vi "Ysingle.vi"(8 "error in (no error)":errorcluster, 11 "MagSpecCamera in":refnum<class "MagSpecCamera.lvclass">) -> (0 "error out":errorcluster, 3 "MagSpecCamera in":refnum<class "MagSpecCamera.lvclass">)   [LabVIEW 2020, in "MagSpecCamera.lvclass"]
uses:
  MagSpecCamera.lvclass
  finalCalib--Cluster.ctl
  MagSpecCamera.lvclass/MagSpecCamera.ctl
  NI_AALBase.lvlib
panel:
  out "Working":i32[](array[numeric])
  out "GOOD - not working":i32[](array[numeric])
  out "pixel angle (y)(pixel)":dbl[][](graph)
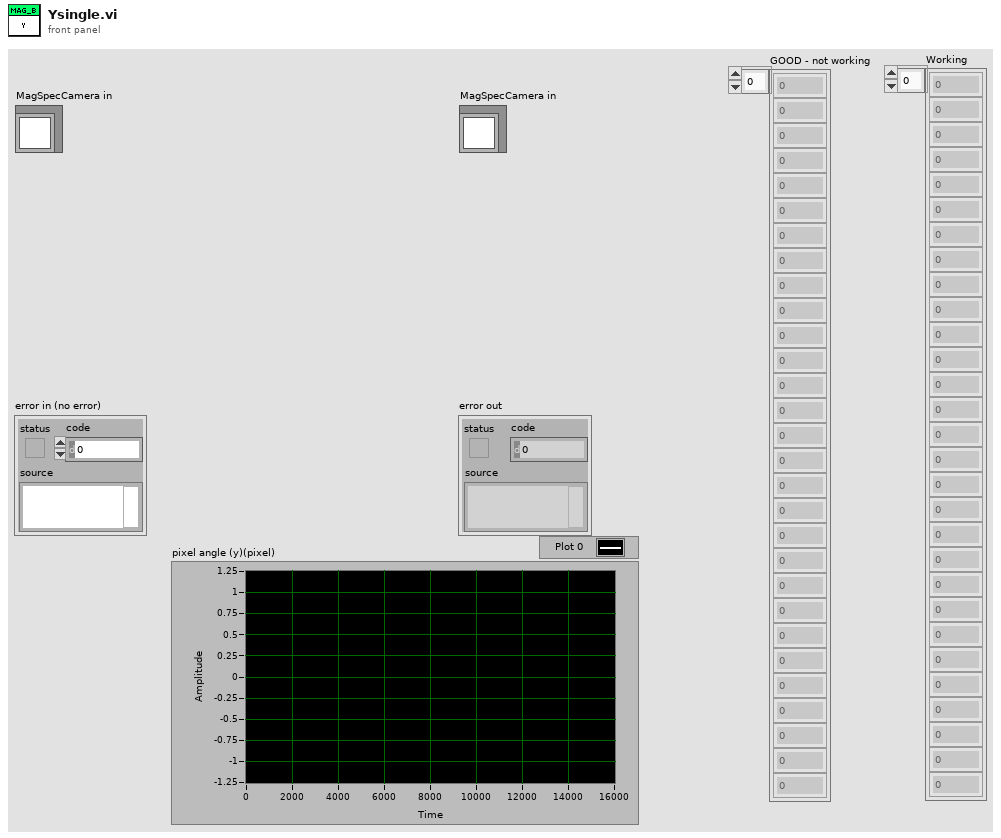
[diagram p1: front panel]
types:
  T1 = typedef "finalCalib--Cluster.ctl" = cluster{"X":dbl[][], "xi":dbl[][], "delta momentum":dbl, "Y":dbl[][], "yi":dbl[][], "angle (Y)":dbl[], "delta angle":dbl, "scale delta angle":dbl, "intraX":dbl, "intraY":dbl, "mask":dbl[][]}
  T2 = typedef "Calibration_Pixel_based.ctl" = cluster{"y1(pixel)":dbl[], "y2(pixel)":dbl[], "dp/B [MeV/C/B] (pixel)":dbl[], "energyDependence Input(pixel)":dbl[], "bending angle [deg](pixel)":dbl[], "total path(pixel)":dbl[], "pixel angle (y)(pixel)":dbl[], "energy dependence (pixel)":dbl[], "charge compensation (pixel)":dbl[], "Momentum [MeV/C](pixel)":dbl[], "angular compensation(pixel)":dbl[]}
  T3 = typedef "CameraSettings_File.ctl" = cluster{"FOV [mm]":dbl, "Left edge [mm]":dbl, "ROI Y offset":dbl, "ROI height":dbl, "ROI X offset":dbl, "ROI width":dbl, "Y center pixel":dbl, "Y Start":dbl, "Y End":dbl, "X Start":dbl, "X End":dbl, "rot [deg]":dbl}
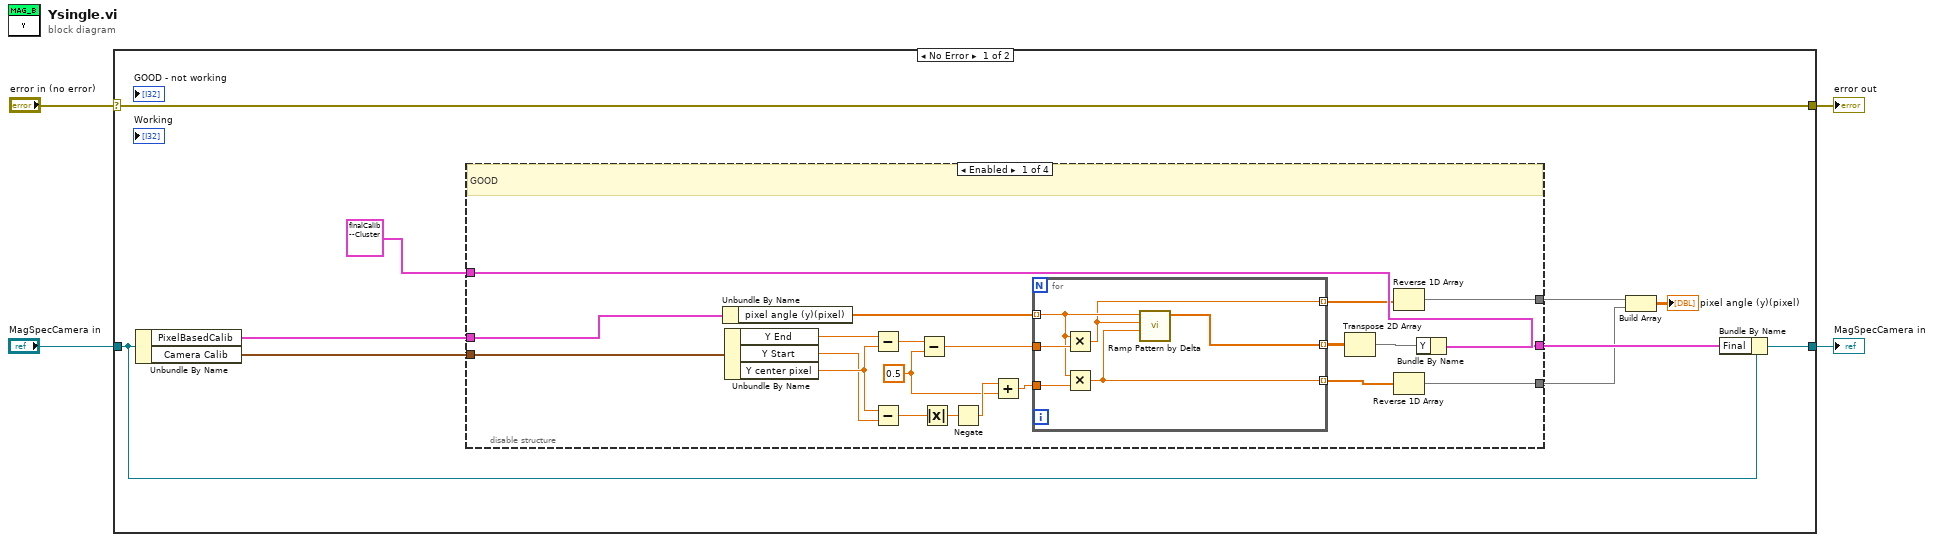
[diagram p0: block diagram]
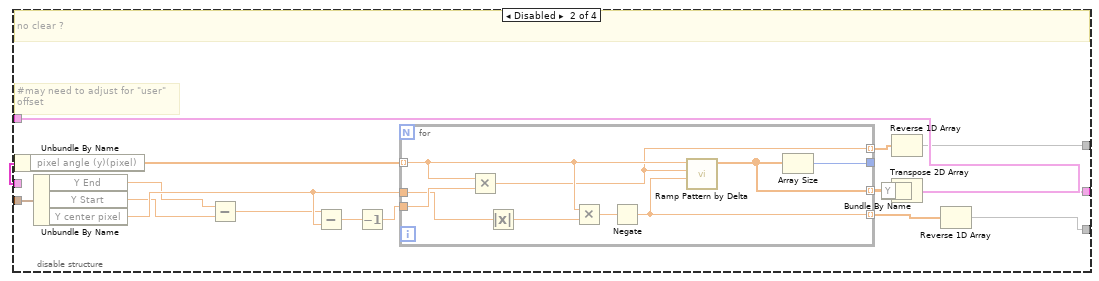
[diagram p2: hidden frame]
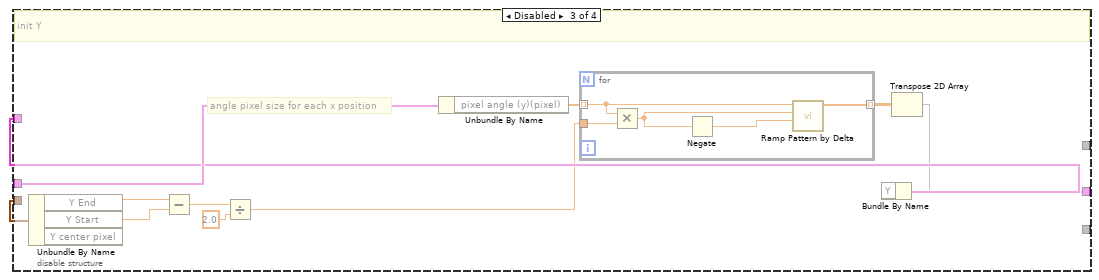
[diagram p3: hidden frame]
diagram:
  n1 = case shown="No Error" "error in (no error)" {
    selector: "error in (no error)" -> [w14 w87]
    tunnel: [w14 w87] -> w3
    tunnel: [w11 w86] -> w1
    tunnel: "MagSpecCamera in" -> [w12 w86]
    frame No Error {
      n2 = Unbundle By Name(w12) -> ("PixelBasedCalib"=w6:T2, "Camera Calib"=w10:T3)
      n3 = disable-structure shown="Enabled" {
        disable-tunnel: w6 -> [w34 w58 w79 _]
        disable-tunnel: T1 {"X"=[], "xi"=[], "delta momentum"=0.0, "Y"=[], "yi"=[], "angle (Y)"=[], "delta angle"=0.0, "scale delta angle"=0.0, "intraX"=0.0, "intraY"=0.0, "mask"=[]} ("Cluster") -> [w33 w57 w77 _]
        disable-tunnel: [w31 w55 w75 _] -> w13
        disable-tunnel: w10 -> [w30 w54 w74 _]
        disable-tunnel: [w27 w47 _ _] -> w9
        disable-tunnel: [w26 w46 _ _] -> w8
        frame Enabled {
          w16 = 0.5
          # "GOOD"
          n4 = Unbundle By Name(w34) -> ("pixel angle (y)(pixel)"=w28:dbl[])
          n5 = Unbundle By Name(w30) -> ("Y End"=w29:dbl, "Y Start"=w24:dbl, "Y center pixel"=w25:dbl)
          n6 = Subtract(x=w29, y=w25) -> (x-y=w19:dbl)
          n7 = Subtract(x=w25, y=w24) -> (x-y=w23:dbl)
          n8 = Subtract(x=w19, y=w16) -> (x-y=w18:dbl)
          n9 = Absolute Value(x=w23) -> (abs(x)=w22:dbl)
          n10 = Negate(x=w22) -> (-x=w17:dbl)
          n11 = Add(x=w17, y=w16) -> (x+y=w15:dbl)
          n12 = for {
            tunnel: w28 -> [w38] mode=indexing
            tunnel: [w41] -> w35 mode=indexing
            tunnel: w18 -> [w40]
            tunnel: w15 -> [w39]
            tunnel: [w37] -> w21 mode=indexing
            tunnel: [w36] -> w20 mode=indexing
            n13 = Multiply(x=w38, y=w40) -> (x*y=w37:dbl)
            n14 = Multiply(x=w38, y=w39) -> (x*y=w36:dbl)
            n15 = call "Ramp Pattern by Delta.vi"("start"=w36, "end"=w37, "delta"=w38) -> ("Ramp Pattern"=w41:dbl[])  [unwired: 6 in, 2 out]
          }
          n16 = Transpose 2D Array(2D array=w35) -> (transposed array=w32:dbl[][])
          n17 = Reverse 1D Array(array=w21) -> (reversed array=w26:dbl[])
          n18 = Reverse 1D Array(array=w20) -> (reversed array=w27:dbl[])
          n19 = Bundle By Name(cluster=w33, "Y"=w32) -> (w31:T1)
        }
        frame Disabled {
          # "#may need to adjust for \"user\"\noffset"
          # "no clear ?"
          n20 = Unbundle By Name(w58) -> ("pixel angle (y)(pixel)"=w50:dbl[])
          n21 = Unbundle By Name(w54) -> ("Y End"=w52:dbl, "Y Start"=w43:dbl, "Y center pixel"=w53:dbl)
          n22 = Subtract(x=w52, y=w43) -> (x-y=w51:dbl)
          n23 = Subtract(x=w51, y=w53) -> (x-y=w45:dbl)
          n24 = Decrement(x=w45) -> (x-1=w44:dbl)
          n25 = for {
            tunnel: w50 -> [w64] mode=indexing
            tunnel: [w61] -> w59 mode=indexing
            tunnel: w44 -> [w68]
            tunnel: w53 -> [w67]
            tunnel: [w63] -> w49 mode=indexing
            tunnel: [w62] -> w48 mode=indexing
            tunnel: [w60] -> w42
            n26 = Multiply(x=w64, y=w68) -> (x*y=w62:dbl)
            n27 = Absolute Value(x=w67) -> (abs(x)=w66:dbl)
            n28 = Multiply(x=w64, y=w66) -> (x*y=w65:dbl)
            n29 = Negate(x=w65) -> (-x=w63:dbl)
            n30 = call "Ramp Pattern by Delta.vi"("start"=w63, "end"=w62, "delta"=w64) -> ("Ramp Pattern"=w61:dbl[])  [unwired: 6 in, 2 out]
            n31 = Array Size(array=w61) -> (size(s)=w60:i32)
          }
          n32 = Reverse 1D Array(array=w48) -> (reversed array=w46:dbl[])
          n33 = Transpose 2D Array(2D array=w59) -> (transposed array=w56:dbl[][])
          n34 = Bundle By Name(cluster=w57, "Y"=w56) -> (w55:T1)
          n35 = Reverse 1D Array(array=w49) -> (reversed array=w47:dbl[])
        }
        frame Disabled {
          # "angle pixel size for each x position"
          # "init Y"
          n36 = Unbundle By Name(w74) -> ("Y End"=w73:dbl, "Y Start"=w72:dbl)  [unwired: 1 out]
          n37 = Subtract(x=w73, y=w72) -> (x-y=w71:dbl)
          n38 = Divide(x=w71, y=2.0) -> (x/y=w69:dbl)
          n39 = Unbundle By Name(w79) -> ("pixel angle (y)(pixel)"=w78:dbl[])
          n40 = for {
            tunnel: w78 -> [w84] mode=indexing
            tunnel: [w85] -> w80 mode=indexing
            tunnel: w69 -> [w83]
            n41 = Multiply(x=w84, y=w83) -> (x*y=w81:dbl)
            n42 = Negate(x=w81) -> (-x=w82:dbl)
            n43 = call "Ramp Pattern by Delta.vi"("start"=w82, "end"=w81, "delta"=w84) -> ("Ramp Pattern"=w85:dbl[])  [unwired: 6 in, 2 out]
          }
          n44 = Transpose 2D Array(2D array=w80) -> (transposed array=w76:dbl[][])
          n45 = Bundle By Name(cluster=w77, "Y"=w76) -> (w75:T1)
        }
        frame Disabled {
        }
      }
      n46 = Build Array(w8, w9) -> (→"pixel angle (y)(pixel)":dbl[][])
      n47 = Bundle By Name(cluster=w12, "Final"=w13) -> (w11:refnum<class "MagSpecCamera.lvclass">)
    }
    frame Error {
    }
  }
  "error out" <- w3
  "MagSpecCamera in" <- w1
